vi "Destroy Request Events.vi"(8 "error in":errorcluster) -> (0 "error out":errorcluster)   [LabVIEW 2024, in "Message.lvlib"]
doc: "Destroy the requests user events, even if there is an incoming error.\n\n<b>NOTE</b>: The contents of this VI are automatically generated and modified by the <b>Tools > DQMH Consortium > DQMH</b> utilities. Consider using those utilities instead of making your own modifications to this VI.\n_____\nBased on DQMH Dev Tools: Project Template 7.1.0.1503."
uses:
  Message.lvlib
panel:
  # "NOTE: The contents of this VI are automatically generated and modified by the Tools > DQMH Consortium > DQMH utilities. Consider using those utilities instead of making your own modifications to this VI."
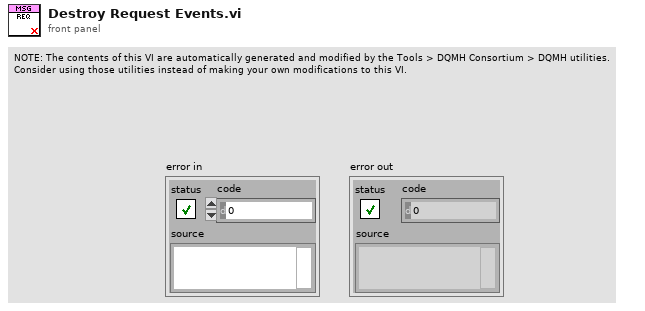
[diagram p1: front panel]
types:
  T1 = typedef "Message.lvlib/Request Events--cluster.ctl" = cluster{"Stop Module":refnum<user-event>, "Show Panel":refnum<user-event>, "Hide Panel":refnum<user-event>, "Show Diagram":refnum<user-event>, "Get Module Execution Status":refnum<user-event>, "Draw FP in Subpanel":refnum<user-event>, "Remove From Subpanel":refnum<user-event>, "Set Message":refnum<user-event>, "Append String":refnum<user-event>, "Set Text Font Settings":refnum<user-event>}
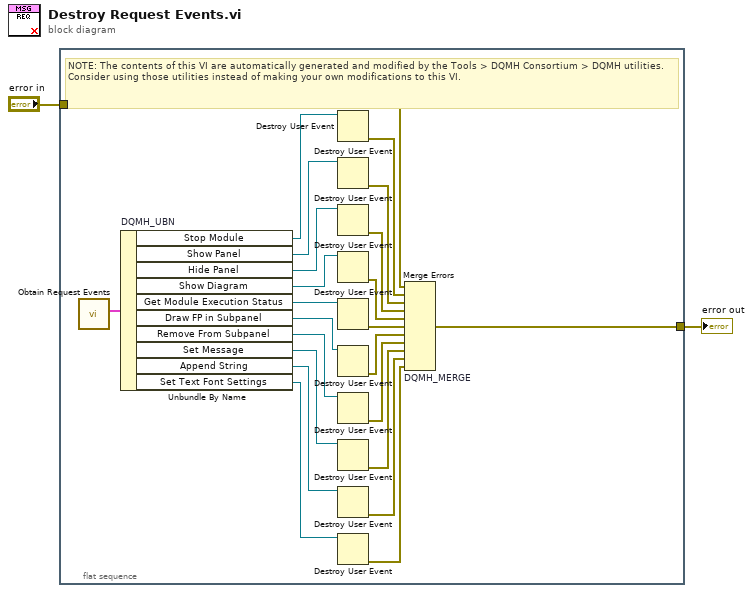
[diagram p0: block diagram]
diagram:
  n1 = flat-sequence {
    tunnel: [w24] -> w2
    tunnel: "error in" -> [w17]
    frame #0 {
      # "NOTE: The contents of this VI are automatically generated and modified by the Tools > DQMH Consortium > DQMH utilities. Consider using those utilities instead of making your own modifications to this VI."
      n2 = call "Obtain Request Events.vi"() -> ("Message Request Events"=w23:T1)  [unwired: 10 in, 1 out]
      n3 = Unbundle By Name "DQMH_UBN"(w23) -> ("Stop Module"=w22:refnum<user-event>, "Show Panel"=w19:refnum<user-event>, "Hide Panel"=w18:refnum<user-event>, "Show Diagram"=w15:refnum<user-event>, "Get Module Execution Status"=w13:refnum<user-event>, "Draw FP in Subpanel"=w11:refnum<user-event>, "Remove From Subpanel"=w9:refnum<user-event>, "Set Message"=w7:refnum<user-event>, "Append String"=w5:refnum<user-event>, "Set Text Font Settings"=w3:refnum<user-event>)
      n4 = Destroy User Event(user event=w22) -> (error out=w25:errorcluster)  [unwired: 1 in]
      n5 = Destroy User Event(user event=w19) -> (error out=w21:errorcluster)  [unwired: 1 in]
      n6 = Destroy User Event(user event=w18) -> (error out=w20:errorcluster)  [unwired: 1 in]
      n7 = Destroy User Event(user event=w15) -> (error out=w16:errorcluster)  [unwired: 1 in]
      n8 = Destroy User Event(user event=w13) -> (error out=w14:errorcluster)  [unwired: 1 in]
      n9 = Destroy User Event(user event=w11) -> (error out=w12:errorcluster)  [unwired: 1 in]
      n10 = Destroy User Event(user event=w9) -> (error out=w10:errorcluster)  [unwired: 1 in]
      n11 = Destroy User Event(user event=w7) -> (error out=w8:errorcluster)  [unwired: 1 in]
      n12 = Destroy User Event(user event=w5) -> (error out=w6:errorcluster)  [unwired: 1 in]
      n13 = Destroy User Event(user event=w3) -> (error out=w4:errorcluster)  [unwired: 1 in]
      n14 = Merge Errors "DQMH_MERGE"(w17, w25, w21, w20, w16, w14, w12, w10, w8, w6, w4) -> (w24:errorcluster)
    }
  }
  "error out" <- w2
